vi "FTW-ScheduledJobset-Find.vi"(0 "FTW Scheduled Jobset":refnum<class "FTW-ScheduledJob.lvclass">[](array[class]), 5 "Identity":string, 11 "error in":errorcluster) -> (4 "FTW Scheduled Jobset out":refnum<class "FTW-ScheduledJob.lvclass">[](array[class]), 6 "Found?":bool, 8 "Index":i32=-1, 15 "error out":errorcluster)   [LabVIEW 2015, in "FTW-ScheduledJob.lvclass"]
uses:
  FTW-ScheduledJob.lvclass
  FTW-ScheduledJob.lvclass/FTW-ScheduledJob.ctl
panel:
  # "Inputs"
  # "Outputs"
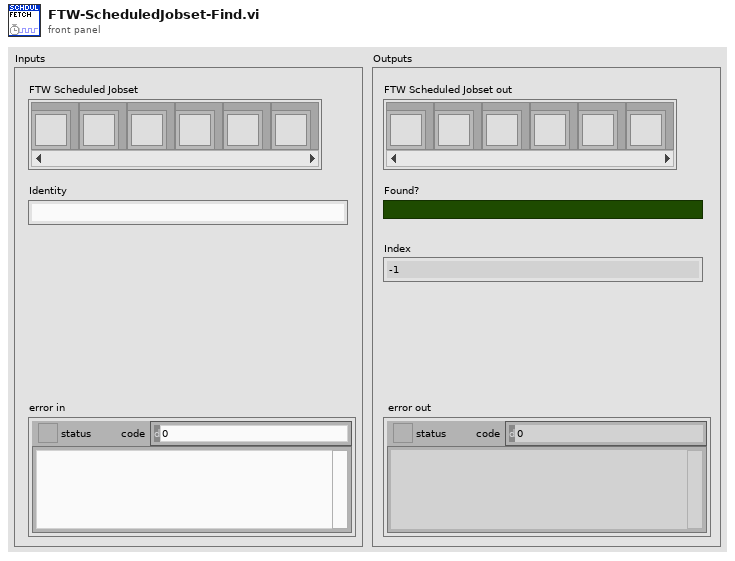
[diagram p1: front panel]
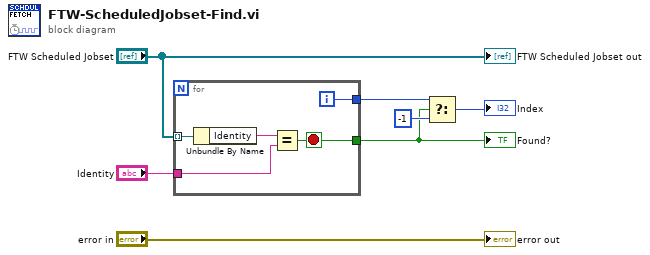
[diagram p0: block diagram]
diagram:
  n1 = for {
    tunnel: "FTW Scheduled Jobset" -> [w12] mode=indexing
    tunnel: "Identity" -> [w10]
    tunnel: [w9] -> w1
    tunnel: [w8] -> w4
    i -> [w8]
    stop <- w9 stop-if-true
    n2 = Unbundle By Name(w12) -> ("Identity"=w11:string)
    n3 = Equal?(x=w11, y=w10) -> (x = y?=w9:bool)
  }
  "Found?" <- w1
  n4 = Select(t=w4, s=w1, f=-1) -> (s? t:f=→"Index":i32)
  "FTW Scheduled Jobset out" <- "FTW Scheduled Jobset"
  "error out" <- "error in"
